vi "Grabold.vi"(6 "AccqMotorRef":T1={"DeviceStatus"={"status"=FALSE, "code"=0, "source"=""}, "Type"=enum."PWM", "PWM"={"Digital Module"=enum."Digital Module 1", "PWM Channel"=enum."Invalid", "DeadBand"={"Name"="", "maxPositivePwm"=0, "minPositivePwm"=0, "centerPwm"=0, "maxNegativePwm"=0, "minNegativePwm"=0, "angularRange"=0}}, "CAN"={"Device Number"=0, "Control Mode"=enum."Percent VBus", "Semaphore"=refnum, "Max Vout"=12.0}, "Invert"=FALSE, "TransformRef"=refnum, "InvTransformRef"=refnum}, 7 "ShoulderMotor":T1={"DeviceStatus"={"status"=FALSE, "code"=0, "source"=""}, "Type"=enum."PWM", "PWM"={"Digital Module"=enum."Digital Module 1", "PWM Channel"=enum."Invalid", "DeadBand"={"Name"="", "maxPositivePwm"=0, "minPositivePwm"=0, "centerPwm"=0, "maxNegativePwm"=0, "minNegativePwm"=0, "angularRange"=0}}, "CAN"={"Device Number"=0, "Control Mode"=enum."Percent VBus", "Semaphore"=refnum, "Max Vout"=12.0}, "Invert"=FALSE, "TransformRef"=refnum, "InvTransformRef"=refnum}) -> ()   [LabVIEW 2013]
uses:
  <vilib>/Rock Robotics/WPI/MotorControl/WPI_MotorControlDeviceRef.ctl
  <vilib>/Rock Robotics/SystemInterfaces/Typedef/FPGA_TypedefDigitalModule.ctl
  <vilib>/Rock Robotics/SystemInterfaces/DIO/FPGA_DIOPWMChannel.ctl
  <vilib>/Rock Robotics/WPI/PWM/WPI_PWMDeadband.ctl
  <vilib>/Rock Robotics/WPI/CAN/Jaguar/SubVIs/WPI_CANJaguar_ControlMode.ctl
  <vilib>/Rock Robotics/WPI/PWM/WPI_PWMTransform_ConPane.ctl
  Events.vi
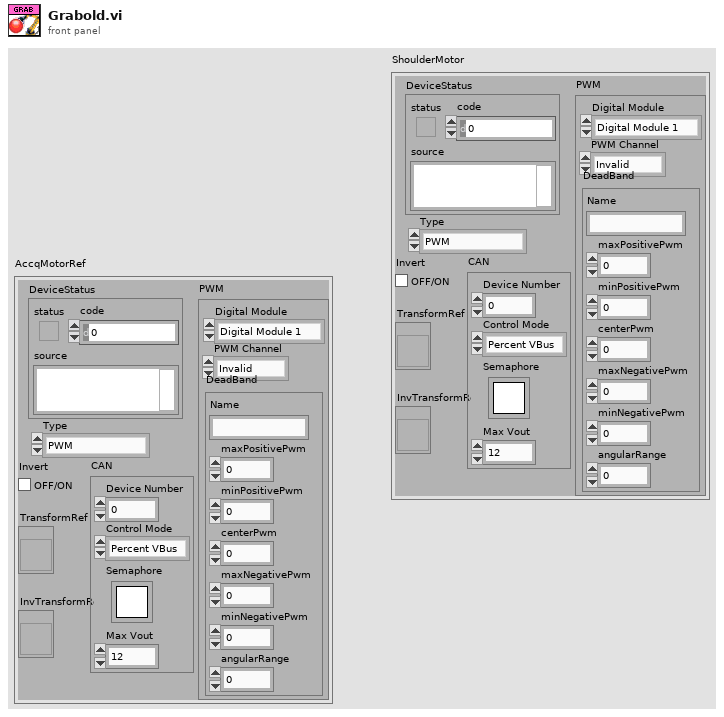
[diagram p1: front panel]
types:
  T1 = typedef "WPI_MotorControlDeviceRef.ctl" = cluster{"DeviceStatus":errorcluster, "Type":enum16{"PWM", "CAN"}, "PWM":cluster{"Digital Module":T2, "PWM Channel":T3, "DeadBand":T4}, "CAN":cluster{"Device Number":u8, "Control Mode":T5, "Semaphore":T6, "Max Vout":dbl}, "Invert":bool, "TransformRef":T7, "InvTransformRef":T7}
  T2 = typedef "FPGA_TypedefDigitalModule.ctl" = enum16{"Digital Module 1", "Digital Module 2"}
  T3 = typedef "FPGA_DIOPWMChannel.ctl" = enum8{"PWM 1", "PWM 2", "PWM 3", "PWM 4", "PWM 5", "PWM 6", "PWM 7", "PWM 8", "PWM 9", "PWM 10", "Invalid"}
  T4 = typedef "WPI_PWMDeadband.ctl" = cluster{"Name":string, "maxPositivePwm":i32, "minPositivePwm":i32, "centerPwm":i32, "maxNegativePwm":i32, "minNegativePwm":i32, "angularRange":u16}
  T5 = typedef "WPI_CANJaguar_ControlMode.ctl" = enum8{"Percent VBus", "Current", "Speed", "Position", "Voltage"}
  T6 = typedef "Semaphore RefNum" = refnum<k1>
  T7 = typedef "WPI_PWMTransform_ConPane.ctl" = refnum<vi>
  T8 = typedef "Eventgrab.ctl" = cluster{"Grab":bool, "GroundPass":bool, "Test Aqaure":dbl, "Shoulder up or down?":bool}
  T9 = typedef "WPI_SolenoidValue.ctl" = enum16{"Off", "On", "Forward", "Reverse"}
  T10 = cluster{"Ultrasonic Distance (In)":dbl, "Gyro":dbl, "TopAquisition sensor":bool, "Encoder distance":dbl, "Encoder rate":dbl, "Encoder direction":bool, "winch engaged?":T9, "Motor Values":dbl[], "Latch encoder":u32, "BottomAquistion":bool}
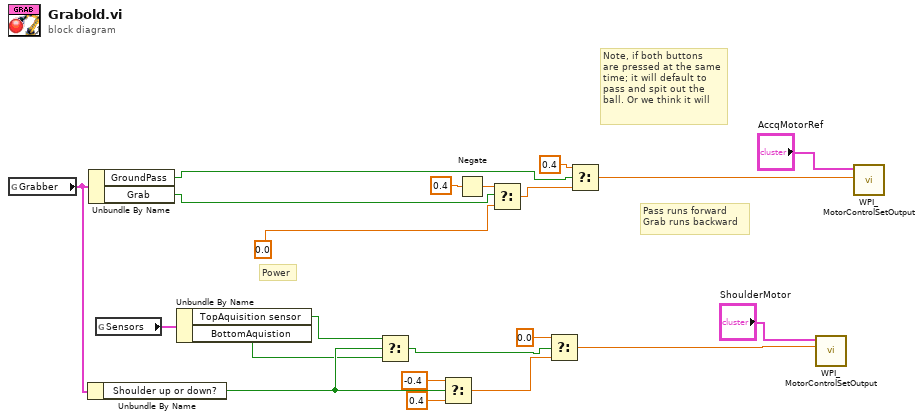
[diagram p0: block diagram]
diagram:
  # "Pass runs forward\nGrab runs backward"
  # "Note, if both buttons\nare pressed at the same\ntime; it will default to\npass and spit out the\nball. Or we think it will"
  # "Power"
  n1 = global read "Events.vi" "Grabber"() -> (w13:T8)
  n2 = Unbundle By Name(w13) -> ("Shoulder up or down?"=w7:bool)
  n3 = Unbundle By Name(w13) -> ("GroundPass"=w17:bool, "Grab"=w18:bool)
  n4 = global read "Events.vi" "Sensors"() -> (w6:T10)
  n5 = Unbundle By Name(w6) -> ("TopAquisition sensor"=w5:bool, "BottomAquistion"=w4:bool)
  n6 = Select(t=w5, s=w7, f=w4) -> (s? t:f=w3:bool)
  n7 = Select(t=-0.4, s=w7, f=0.4) -> (s? t:f=w8:dbl)
  n8 = Negate(x=0.4 ("Power")) -> (-x=w19:dbl)
  n9 = Select(t=w19, s=w18, f=0.0) -> (s? t:f=w20:dbl)
  n10 = Select(t=0.0, s=w3, f=w8) -> (s? t:f=w12:dbl)
  n11 = Select(t=0.4, s=w17, f=w20) -> (s? t:f=w14:dbl)
  n12 = call <vilib>:"WPI_MotorControlSetOutput.vi"("Output"=w12, "MotorControlDevRef"="ShoulderMotor") -> ()  [unwired: 7 in, 3 out]
  n13 = call <vilib>:"WPI_MotorControlSetOutput.vi"("Output"=w14, "MotorControlDevRef"="AccqMotorRef") -> ()  [unwired: 7 in, 3 out]
